vi "Motor_Pos_from_GlobaL_Variable.vi"(9 "Motor":u16(ring)=2 items=["none", "1", "2", "3", "4", "all"], 11 "Manipulator Pos IN":i32[](array[numeric])) -> (1 "Motor Index":i32, 3 "Motor Pos":i32)   [LabVIEW 2018]
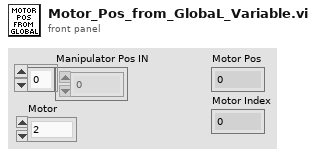
[diagram p1: front panel]
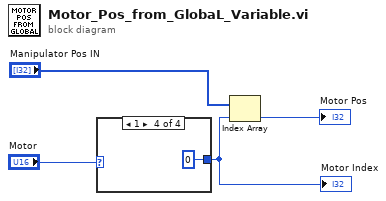
[diagram p0: block diagram]
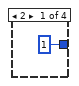
[diagram p2: hidden frame]
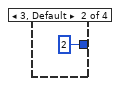
[diagram p3: hidden frame]
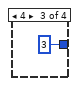
[diagram p4: hidden frame]
diagram:
  n1 = case shown="1" "Motor" {
    tunnel: [1 2 3 0] -> w2
    frame 2 {
    }
    frame 3, Default {
    }
    frame 4 {
    }
    frame 1 {
    }
  }
  "Motor Index" <- w2
  n2 = Index Array(array="Manipulator Pos IN", index=w2) -> (element=→"Motor Pos":i32)
